vi "SR830ReadOutInputs.vi"(0 "VISA resource name":refnum<visa-resource-name>, 11 "error in (no error)":errorcluster) -> (4 "VISA resource name out":refnum<visa-resource-name>, 12 "R":dbl, 13 "Theta":dbl, 14 "Aux In 1":dbl, 15 "error out":errorcluster)   [LabVIEW 2016]
uses:
  <instrlib>/Stanford Research 830/Stanford Research 830.lvlib
panel:
  # "This VI reads out R, Theta, and Aux In 1 simulataneously."
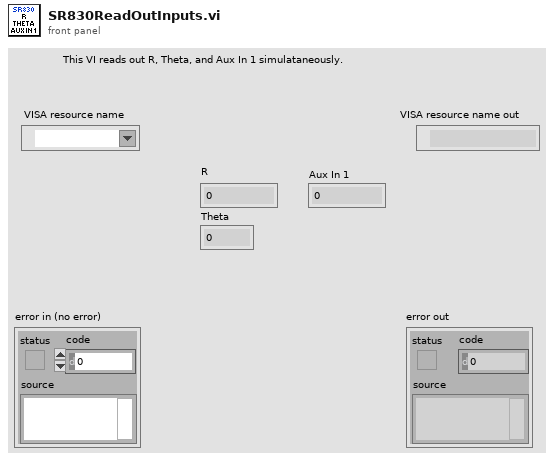
[diagram p1: front panel]
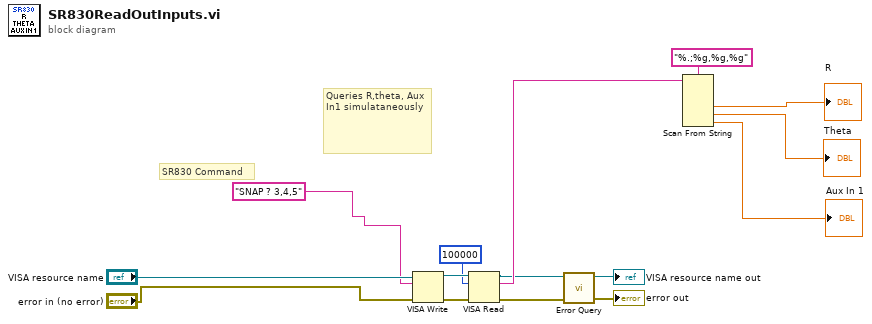
[diagram p0: block diagram]
diagram:
  # "SR830 Command"
  # "Queries R,theta, Aux In1 simulataneously"
  n1 = VISA Write(VISA resource name="VISA resource name", write buffer="SNAP ? 3,4,5", error in (no error)="error in (no error)") -> (VISA resource name out=w14:refnum<visa-resource-name>, error out=w15:errorcluster)  [unwired: 1 out]
  n2 = VISA Read(VISA resource name=w14, byte count=u32 100000, error in (no error)=w15) -> (VISA resource name out=w5:refnum<visa-resource-name>, read buffer=w9:string, error out=w6:errorcluster)  [unwired: 1 out]
  n3 = call <instrlib>:"Error Query.vi"("error in (no error)"=w6, "VISA resource name"=w5) -> ("error out"=→"error out":errorcluster, "VISA resource name out"=→"VISA resource name out":refnum<visa-resource-name>)  [unwired: 7 in, 1 out]
  n4 = Scan From String(format string="%.;%g,%g,%g", input string=w9) -> (output 1=→"R":dbl, output 2=→"Theta":dbl, output 3=→"Aux In 1":dbl)  [unwired: 5 in, 3 out]
